vi "Platform Specific Directory Separator.vi"() -> (3 "search string":string)   [LabVIEW 2020, in "Test Finder.lvclass"]
uses:
  Test Finder.lvclass
  Test Finder.lvclass/Test Finder.ctl
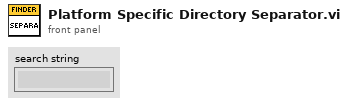
[diagram p1: front panel]
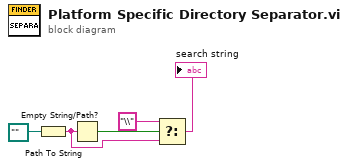
[diagram p0: block diagram]
diagram:
  n1 = Path To String(path=path "") -> (string=w4:string)
  n2 = Empty String/Path?(string/path=w4) -> (empty?=w2:bool)
  n3 = Select(t="\\" ("search string"), s=w2, f=w4) -> (s? t:f=→"search string":string)
